vi "cRIO_4DoF_Fsense_deadband(subVI).vi"(9 "Fsense deadband (Nm or N)":dbl[](array[numeric]), 10 "Enable Fsense Deadband":bool, 11 "F_{2} in":dbl[](array[numeric])) -> (3 "F_{2} out":dbl[](array[numeric]))   [LabVIEW 2019]
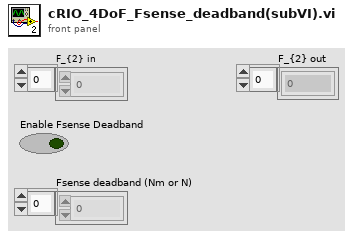
[diagram p1: front panel]
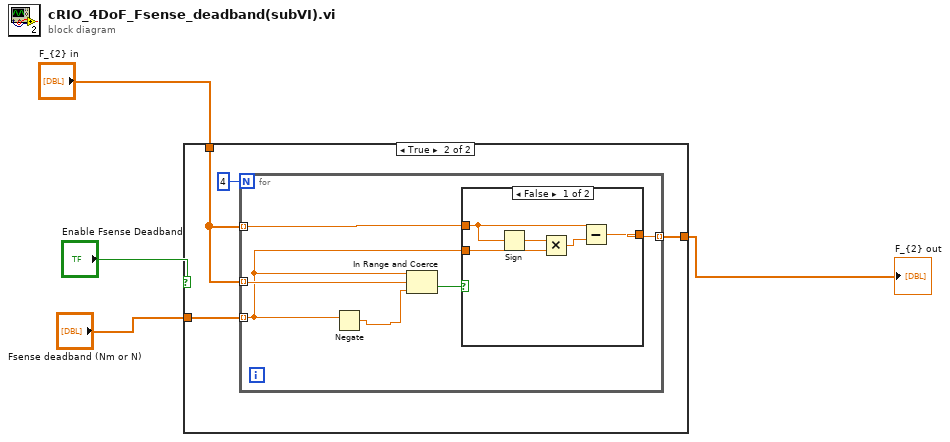
[diagram p0: block diagram]
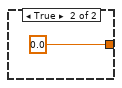
[diagram p3: hidden frame]
diagram:
  n1 = case shown="True" "Enable Fsense Deadband" {
    tunnel: "Fsense deadband (Nm or N)" -> [_ w8]
    tunnel: "F_{2} in" -> [w5 w7]
    tunnel: [w5 w6] -> w4
    frame False {
    }
    frame True {
      n2 = for {
        N: 4 -> [_]
        tunnel: w7 -> [w15] mode=indexing
        tunnel: w8 -> [w10] mode=indexing
        tunnel: [w13] -> w6 mode=indexing
        tunnel: w7 -> [w12] mode=indexing
        n3 = Negate(x=w10) -> (-x=w11:dbl)
        n4 = In Range and Coerce(upper limit=w10, x=w15, lower limit=w11) -> (In Range?=w14:bool)  [unwired: 1 out]
        n5 = case shown="False" w14 {
          tunnel: [w16 0.0] -> w13
          tunnel: w12 -> [w20 _]
          tunnel: w10 -> [w18 _]
          frame False {
            n6 = Sign(1:w20) -> (0:w19:dbl)
            n7 = Multiply(x=w19, y=w18) -> (x*y=w17:dbl)
            n8 = Subtract(x=w20, y=w17) -> (x-y=w16:dbl)
          }
          frame True {
          }
        }
      }
    }
  }
  "F_{2} out" <- w4
